vi "Create Defaults String.vi"(8 "error in (no error)":errorcluster, 9 "Exception Values":string[](array[string]), 10 "Exception Names":string[](array[string]), 11 "Array":refnum<vi>[](array[refnum])) -> (0 "error out":errorcluster, 3 "regular expression":string)   [LabVIEW 2025, in "Tools.lvlib"]
uses:
  Tools.lvlib
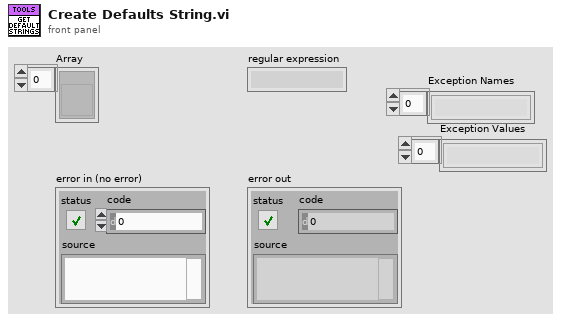
[diagram p1: front panel]
types:
  T1 = typedef "Tools.lvlib/Datatypes.ctl" = enum16{"Float", "Int", "String", "String Array", "Int Array", "Float Array", "Bool Array", "Bool", "Invalid"}
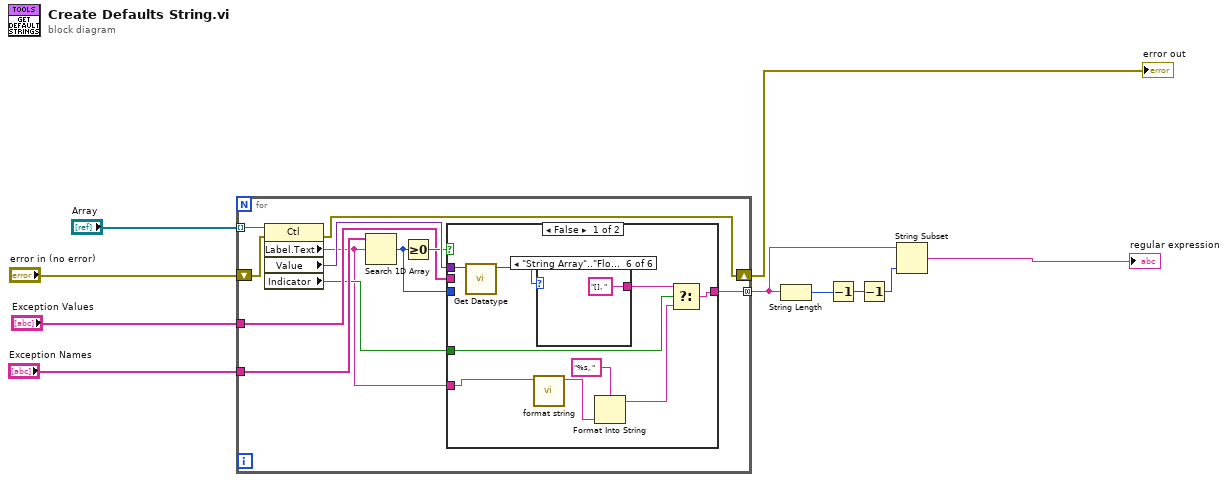
[diagram p0: block diagram]
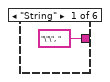
[diagram p2: hidden frame]
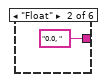
[diagram p3: hidden frame]
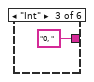
[diagram p4: hidden frame]
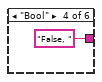
[diagram p5: hidden frame]
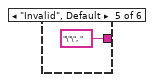
[diagram p6: hidden frame]
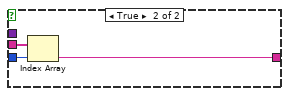
[diagram p7: hidden frame]
diagram:
  n1 = for {
    tunnel: "Array" -> [w20] mode=indexing
    shift-right: [w14] -> w9
    shift-left: "error in (no error)" -> [w21]
    tunnel: [w12] -> w2 mode=concatenating
    tunnel: "Exception Names" -> [w18]
    tunnel: "Exception Values" -> [w16]
    n2 = property class="Ctl"(reference=w20, error in=w21) -> (error out=w14:errorcluster, "Label.Text"=w11:string, "Value"=w19:variant, "Indicator"=w13:bool)  [unwired: 1 out]
    n3 = Search 1D Array(1D array=w18, element=w11) -> (index of element=w15:i32)  [unwired: 1 in]
    n4 = Greater Or Equal To 0?(x=w15) -> (x >= 0?=w17:bool)
    n5 = case shown="False" w17 {
      tunnel: w19 -> [w29 _]
      tunnel: w16 -> [_ w39]
      tunnel: w15 -> [_ w38]
      tunnel: w13 -> [w28 _]
      tunnel: [w26 w37] -> w12
      tunnel: w11 -> [w25 _]
      frame False {
        n6 = call "Get Datatype.vi"("Value"=w29) -> ("datatypes"=w30:T1)  [unwired: 10 in]
        n7 = call "format string.vi"("Label.Text"=w25) -> ("String"=w24:string)  [unwired: 10 in]
        n8 = case shown="\"String Array\"..\"Float Array\"" w30 {
          tunnel: ["\"\", " ("format string") "0.0, " ("format string") "0, " ("format string") "False, " ("format string") "\"\", " ("format string") "[], " ("format string")] -> w27
          frame "String" {
          }
          frame "Float" {
          }
          frame "Int" {
          }
          frame "Bool" {
          }
          frame "Invalid", Default {
          }
          frame "String Array".."Float Array" {
          }
        }
        n9 = Format Into String(format string="%s, ", w24) -> (resulting string=w22:string)  [unwired: 2 in, 1 out]
        n10 = Select(t=w27, s=w28, f=w22) -> (s? t:f=w26:string)
      }
      frame True {
        n11 = Index Array(array=w39, index=w38) -> (element=w37:string)
      }
    }
  }
  "error out" <- w9
  n12 = String Length(string=w2) -> (length=w4:i32)
  n13 = Decrement(x=w4) -> (x-1=w3:i32)
  n14 = Decrement(x=w3) -> (x-1=w5:i32)
  n15 = String Subset(string=w2, length (rest)=w5) -> (substring=→"regular expression":string)  [unwired: 1 in]
